vi "Agilent 681x Custom Waveform Output.vi"() -> ()   [LabVIEW 2019]
doc: "Demonstrates how a custom waveform should be created and be used for output."
uses:
  <instrlib>/Agilent 681x Series/Agilent 681x Series.lvlib
panel:
  in  "Output Frequency (60 Hz)":dbl=60.0 format="%#.4g"
  in  "Voltage Amplitude (1.0 V)":dbl=1.0 format="%#.4g"
  in  "Waveform Values":dbl[](array[numeric])=[1.0, 2.0, 3.0, 4.0]
  in  "Waveform Name":string
  in  "Serial Configuration":T1={"Baud Rate"=9600, "Parity"=0, "Data Bits"=7} {"Data Bits" items=["7"=7, "8"=8]; "Parity" items=["None", "Odd", "Even", "Mark", "Space"]; "Baud Rate" items=["300"=300, "600"=600, "1200"=1200, "2400"=2400, "4800"=4800, "9600"=9600]}
  in  "VISA resource name":refnum<visa-resource-name>
  # "(c) 2008-2021 National Instruments Corp.  ALL RIGHTS RESERVED."
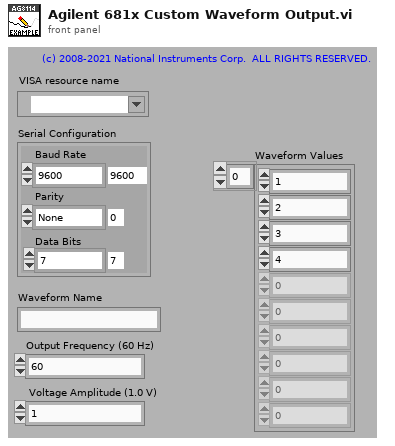
[diagram p1: front panel]
types:
  T1 = cluster{"Baud Rate":u32, "Parity":u16, "Data Bits":u16}
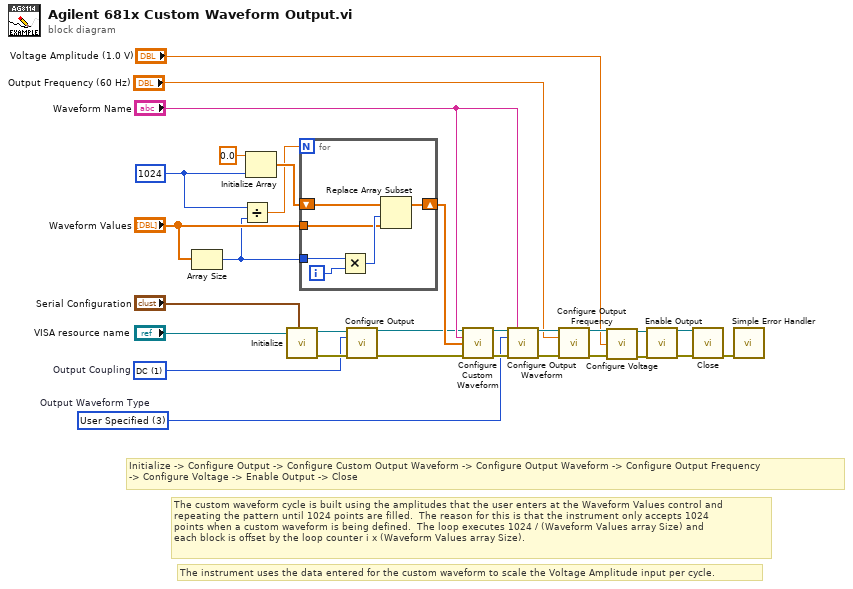
[diagram p0: block diagram]
diagram:
  w14 = 1 items=["AC", "DC"]  # Output Coupling
  w23 = u16 3 items=["Sinusoid", "Square", "Clipped Sinusoid", "User Specified"]  # Output Waveform Type
  w8 = 1024 ("dimension size")
  # "Initialize -> Configure Output -> Configure Custom Output Waveform -> Configure Output Waveform -> Configure Output Frequency\n-> Configure Voltage -> Enable Output -> Close"
  # "The instrument uses the data entered for the custom waveform to scale the Voltage Amplitude input per cycle."
  # "The custom waveform cycle is built using the amplitudes that the user enters at the Waveform Values control and\nrepeating the pattern until 1024 points are filled.  The reason for this is that the instrument only accepts 1024\npoints when a custom waveform is being defined.  The loop executes 1024 / (Waveform Values array Size) and \neach block is offset by the loop counter i x (Waveform Values array Size)."
  n1 = Array Size(array="Waveform Values") -> (size(s)=w6:i32)
  n2 = Divide(x=w8, y=w6) -> (x/y=w9:dbl)
  n3 = Initialize Array(0.0 ("element"), w8) -> (w26:dbl[])
  n4 = call <instrlib>:"Initialize.vi"("Serial Configuration"="Serial Configuration", "VISA resource name"="VISA resource name") -> ("error out"=w17:errorcluster, "VISA resource name out"=w18:refnum<visa-resource-name>)  [unwired: 8 in]
  n5 = for {
    N: w9 -> [_]
    tunnel: "Waveform Values" -> [w31]
    shift-right: [w34] -> w19
    shift-left: w26 -> [w35]
    tunnel: w6 -> [w30]
    i -> [w33]
    n6 = Multiply(x=w30, y=w33) -> (x*y=w32:i32)
    n7 = Replace Array Subset(array=w35, new element=w31, index=w32) -> (w34:dbl[])
  }
  n8 = call <instrlib>:"Configure Output.vi"("VISA resource name"=w18, "Output Coupling (0: AC)"=w14, "error in (no error)"=w17) -> ("VISA resource name out"=w15:refnum<visa-resource-name>, "error out"=w16:errorcluster)  [unwired: 11 in]
  n9 = call <instrlib>:"Configure Custom Waveform.vi"("VISA resource name"=w15, "Waveform Name"="Waveform Name", "Waveform Amplitude Values"=w19, "error in (no error)"=w16) -> ("VISA resource name out"=w25:refnum<visa-resource-name>, "error out"=w24:errorcluster)  [unwired: 10 in]
  n10 = call <instrlib>:"Configure Output Waveform.vi"("VISA resource name"=w25, "User-Specified Output Waveform Name"="Waveform Name", "Output Waveform Type (0: Sinusoid)"=w23, "error in (no error)"=w24) -> ("VISA resource name out"=w20:refnum<visa-resource-name>, "error out"=w21:errorcluster)  [unwired: 10 in]
  n11 = call <instrlib>:"Configure Output Frequency.vi"("VISA resource name"=w20, "Output Frequency (60 Hz)"="Output Frequency (60 Hz)", "error in (no error)"=w21) -> ("VISA resource name out"=w13:refnum<visa-resource-name>, "error out"=w12:errorcluster)  [unwired: 11 in]
  n12 = call <instrlib>:"Configure Voltage.vi"("VISA resource name"=w13, "Voltage Amplitude (1.0 V)"="Voltage Amplitude (1.0 V)", "error in (no error)"=w12) -> ("VISA resource name out"=w10:refnum<visa-resource-name>, "error out"=w11:errorcluster)  [unwired: 11 in]
  n13 = call <instrlib>:"Enable Output.vi"("VISA resource name"=w10, "error in (no error)"=w11) -> ("VISA resource name out"=w4:refnum<visa-resource-name>, "error out"=w5:errorcluster)  [unwired: 12 in]
  n14 = call <instrlib>:"Close.vi"("error in (no error)"=w5, "VISA resource name"=w4) -> ("error out"=w3:errorcluster)  [unwired: 9 in]
  n15 = call <vilib>:"Simple Error Handler.vi"("error in (no error)"=w3) -> ()  [unwired: 4 in, 5 out]
